vi "Read Post-Setup Msgs.vi"(11 "Base Msg Self in":refnum<class "Base Msg Self.lvclass">) -> (2 "Post-Setup Msgs":refnum<class "Msg.lvclass">[](array[class]))   [LabVIEW 2020, in "jettl.lvlib" / "Base Msg Self.lvlib" / "Base Msg Self.lvclass"]
uses:
  Base Msg Self.lvclass
  Base Msg Self.lvclass/Base Msg Self.ctl
  Msg/Msg.lvclass
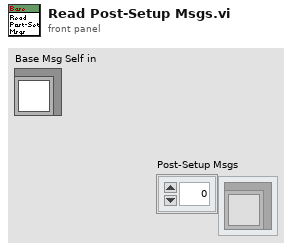
[diagram p1: front panel]
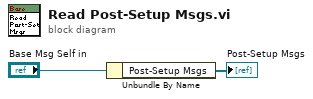
[diagram p0: block diagram]
diagram:
  n1 = Unbundle By Name("Base Msg Self in") -> ("Post-Setup Msgs"=→"Post-Setup Msgs":refnum<class "Msg.lvclass">[])
